vi "GetType.vi"(8 "error in (no error)":errorcluster, 11 "Set Delays Msg":refnum<class "Set Delays Msg.lvclass">) -> (0 "error out":errorcluster, 2 "Data Sample":variant, 3 "Set Delays Msg":refnum<class "Set Delays Msg.lvclass">)   [LabVIEW 2019, in "BNT_DAQmx.lvlib" / "Set Delays Msg.lvclass"]
uses:
  Set Delays Msg.lvclass
  Set Delays Msg.lvclass/Set Delays Msg.ctl
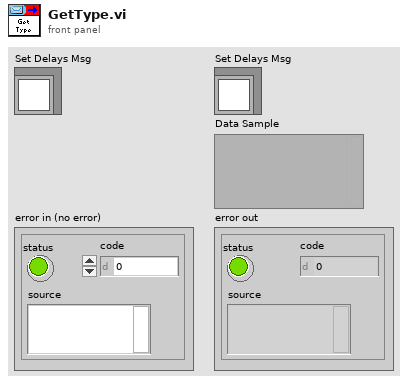
[diagram p1: front panel]
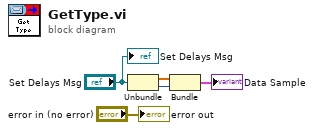
[diagram p0: block diagram]
diagram:
  n1 = Unbundle("Set Delays Msg") -> (w2:dbl[], w1:i32)
  n2 = Bundle("PWM Delays"=w2, "Start Index"=w1) -> (→"Data Sample":cluster{"PWM Delays":dbl[], "Start Index":i32})  [unwired: 1 in]
  "error out" <- "error in (no error)"
  "Set Delays Msg" <- "Set Delays Msg"
